vi "control-logic-sample-4-1.vi"() -> ()   [LabVIEW 2020]
panel:
  out "SYSTEM\nRUN":bool
  in  "PERMISSIVE":bool
  in  "AUTO RUN\nREQUEST":bool
  in  "MANUAL\nUSER RUN\nREQUEST":bool
  in  "AUTO\nMODE":bool
  in  "STOP":bool
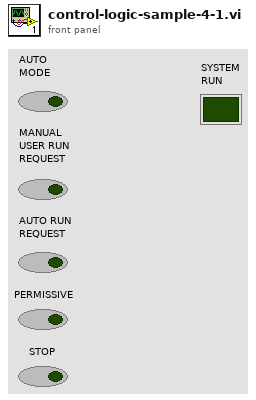
[diagram p1: front panel]
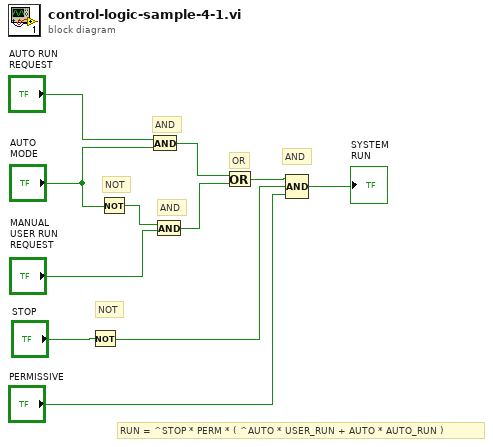
[diagram p0: block diagram]
diagram:
  # "RUN = ^STOP * PERM * ( ^AUTO * USER_RUN + AUTO * AUTO_RUN )"
  # "NOT"
  # "AND"
  # "OR"
  # "NOT"
  # "AND"
  # "AND"
  n1 = Not(x="STOP") -> (.not. x?=w3:bool)
  n2 = Not(x="AUTO\nMODE") -> (.not. x?=w9:bool)
  n3 = And(x="AUTO RUN\nREQUEST", y="AUTO\nMODE") -> (x .and. y?=w7:bool)
  n4 = And(x=w9, y="MANUAL\nUSER RUN\nREQUEST") -> (x .and. y?=w6:bool)
  n5 = Or(x=w7, y=w6) -> (x .or. y?=w5:bool)
  n6 = Compound Arithmetic op=AND(w5, w3, "PERMISSIVE") -> (→"SYSTEM\nRUN":bool)
